vi "CheckName(SubVI).vi"(8 "Error In":errorcluster, 10 "Name In":string, 11 "Strings And Values[]":cluster{"String":string, "Value":string}[](array[cluster])) -> (0 "Error Out":errorcluster, 3 "Name Out":string)   [LabVIEW 2018]
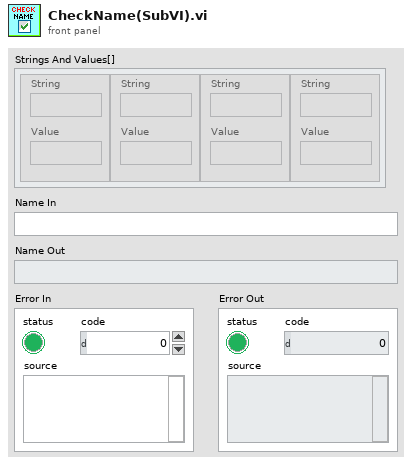
[diagram p1: front panel]
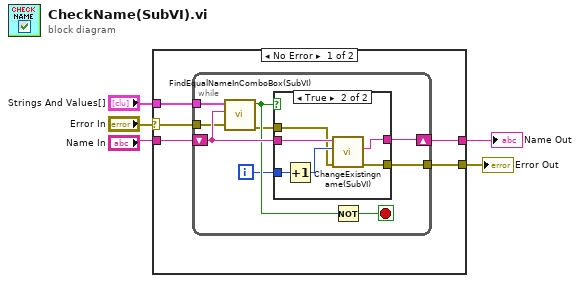
[diagram p0: block diagram]
diagram:
  n1 = case shown="No Error" "Error In" {
    selector: "Error In" -> [w7 w28]
    tunnel: "Strings And Values[]" -> [w10 _]
    tunnel: "Name In" -> [w9 _]
    tunnel: [w8 _] -> w3
    tunnel: [w6 w28] -> w1
    frame No Error {
      n2 = while {
        tunnel: w10 -> [w19]
        shift-right: [w15] -> w8
        shift-left: w9 -> [w18]
        tunnel: w7 -> [w13]
        tunnel: [w11] -> w6
        i -> [w14]
        stop <- w17 stop-if-true
        n3 = call "FindEqualNameInComboBox(SubVI).vi"("Error In"=w13, "Name"=w18, "Strings And Values[]"=w19) -> ("Error Out"=w12:errorcluster, "Does the array contain this name?"=w16:bool)  [unwired: 6 in, 1 out]
        n4 = case shown="True" w16 {
          tunnel: w18 -> [w21 w25]
          tunnel: [w21 w24] -> w15
          tunnel: w14 -> [_ w27]
          tunnel: w12 -> [w20 w23]
          tunnel: [w20 w22] -> w11
          frame False {
          }
          frame True {
            n5 = Increment(x=w27) -> (x+1=w26:i32)
            n6 = call "ChangeExistingname(SubVI).vi"("Error In"=w23, "Numb"=w26, "Name In"=w25) -> ("Error Out"=w22:errorcluster, "Result string"=w24:string)  [unwired: 7 in]
          }
        }
        n7 = Not(x=w16) -> (.not. x?=w17:bool)
      }
    }
    frame Error {
    }
  }
  "Name Out" <- w3
  "Error Out" <- w1
